vi "Actor Core.vi"(8 "error in (no error)":errorcluster, 11 "Simple Actor in":refnum<class "Simple Actor.lvclass">) -> (0 "error out":errorcluster, 3 "Simple Actor out":refnum<class "Simple Actor.lvclass">)   [LabVIEW 2020, in "Simple Actor.lvlib" / "Simple Actor.lvclass"]
uses:
  Simple Actor.lvclass
  Initialize Msg/Initialize Msg.lvclass
  E:/NI I Program/Actor Intr Demo/Simple Actor/Actor Msg/Actor Msg.lvclass
  Simple Actor.lvclass/Simple Actor.ctl
  Actor Msg/Actor Msg.lvclass
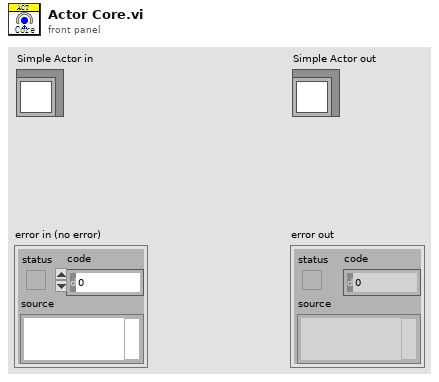
[diagram p1: front panel]
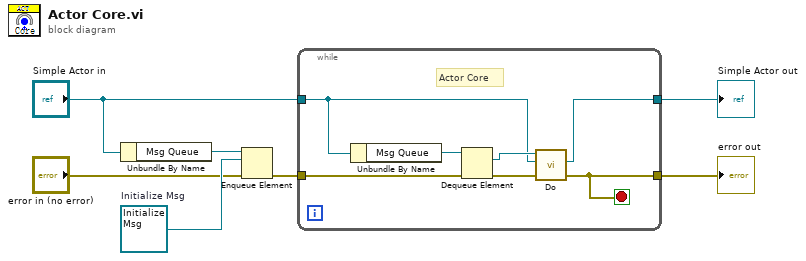
[diagram p0: block diagram]
diagram:
  w3 = refnum<class "Initialize Msg.lvclass"> refnum  # Initialize Msg
  n1 = Unbundle By Name("Simple Actor in") -> ("Msg Queue"=w4:refnum<queue>)
  n2 = Enqueue Element(queue=w4, element=w3, error in (no error)="error in (no error)") -> (error out=w1:errorcluster)  [unwired: 1 in, 2 out]
  n3 = while {
    tunnel: "Simple Actor in" -> [w9]
    tunnel: [w8] -> w7
    tunnel: w1 -> [w11]
    tunnel: [w10] -> w6
    stop <- w10 stop-if-true
    # "Actor Core"
    n4 = Unbundle By Name(w9) -> ("Msg Queue"=w14:refnum<queue>)
    n5 = Dequeue Element(queue=w14, error in (no error)=w11) -> (element=w13:refnum<class "Actor Msg.lvclass">, error out=w12:errorcluster)  [unwired: 1 in, 2 out]
    n6 = call-dynamic "Do.vi"("error in (no error)"=w12, "Actor in"=w9, "Actor Msg in"=w13) -> ("error out"=w10:errorcluster, "Actor out"=w8:refnum<class "Simple Actor.lvclass">)  [unwired: 6 in, 1 out]
  }
  "error out" <- w6
  "Simple Actor out" <- w7
